vi "Config.Global.vi"() -> ()   [LabVIEW 2016]
uses:
  EventLog/EventLog.Gui.Sets.ctl
  EventLog/EventLog.EventLevelOperatorGui.ctl
panel:
  in  "Password":string="9cef32a69bddb65b2d050540c258c086"
  in  "EventModeOptions":T1 caption="Event.Sets" {"dtm_End" format="%<%.1X\n%x>T"; "dtm_Begin" format="%<%.1X\n%x>T"}
  in  "Language":string
  in  "Touchpanel":bool
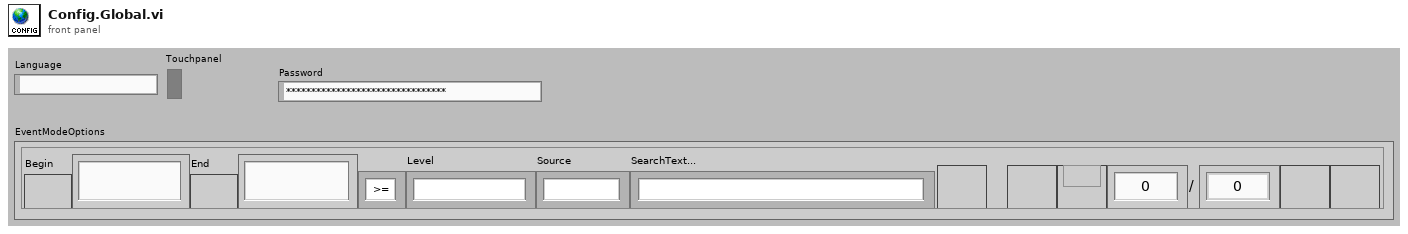
[diagram p1: front panel]
types:
  T1 = typedef "EventLog.Gui.Sets.ctl" = cluster{"IncludeBegin":bool, "dtm_Begin":timestamp, "IncludeEnd":bool, "dtm_End":timestamp, "Events Level Operator":T2, "Level":u16, "Source":u16, "SearchText":string, "Refresh":bool, "Pages":i32, "PageNo":i32, "First":bool, "Prev":bool, "Next":bool, "Last":bool}
  T2 = typedef "EventLog.EventLevelOperatorGui.ctl" = enum16{">=", "=", "<="}
diagram:
